vi "SPI API - SPI Simulation.vi"() -> ()   [LabVIEW 2014]
uses:
  Controls/Timing Characteristics.ctl
  Controls/Digital Data.ctl
  <vilib>/rvi/DesktopExecutionNode/Execution/niFpgaDEN_Execute.vi
  <vilib>/rvi/DesktopExecutionNode/DesktopExecutionNode.xnode
panel:
  in  "SPI PHY Settings":T1={"Divide Value"=10, "Transfer Length (bits)"=16, "CS Asserted Polarity"=FALSE, "Clock Polarity (CPOL)"=FALSE, "Clock Phase (CPHA)"=FALSE, "Lengthen MISO Setup"=FALSE, "Direction Change Bit"=0, "MOSI Starts as Output"=FALSE, "Tristatable MOSI"=FALSE}
  in  "Chip Select":u8
  in  "Engine Rate (MHz)":i32=120
  out "Data To Slave":u64 format="%b"
  out "Timing Characteristics":T2 {"tCL (ns)" format="%#_4g"; "tCH (ns)" format="%#_4g"; "tCSS (ns)" format="%#_4g"; "tCSH (ns)" format="%#_4g"; "tCSW (ns)" format="%#_4g"; "Actual Sample Rate (Hz)" format="%_4p"; "SCLK Frequency (Hz)" format="%#.2p"}
  in  "Pause":bool
  in  "Sample Rate (Hz)":u32=100000 format="%.0p"
  out "Digital Data":digitalwaveform(graph)
  in  "Data To Slave":u64 format="%x"
  in  "Stop":bool
  # "Operating Instructions\n1. For this VI to work, the FPGA must be in Simulation Mode.\n2. Set the 'Engine Rate' control value to match your FPGA SPI Engine loop rate.\n3. Select a sample rate to control how often the SPI message is transmitted.\n4. Run the VI and observe the Timing Characterstics to the right."
  # "Typical Timing Diagram"
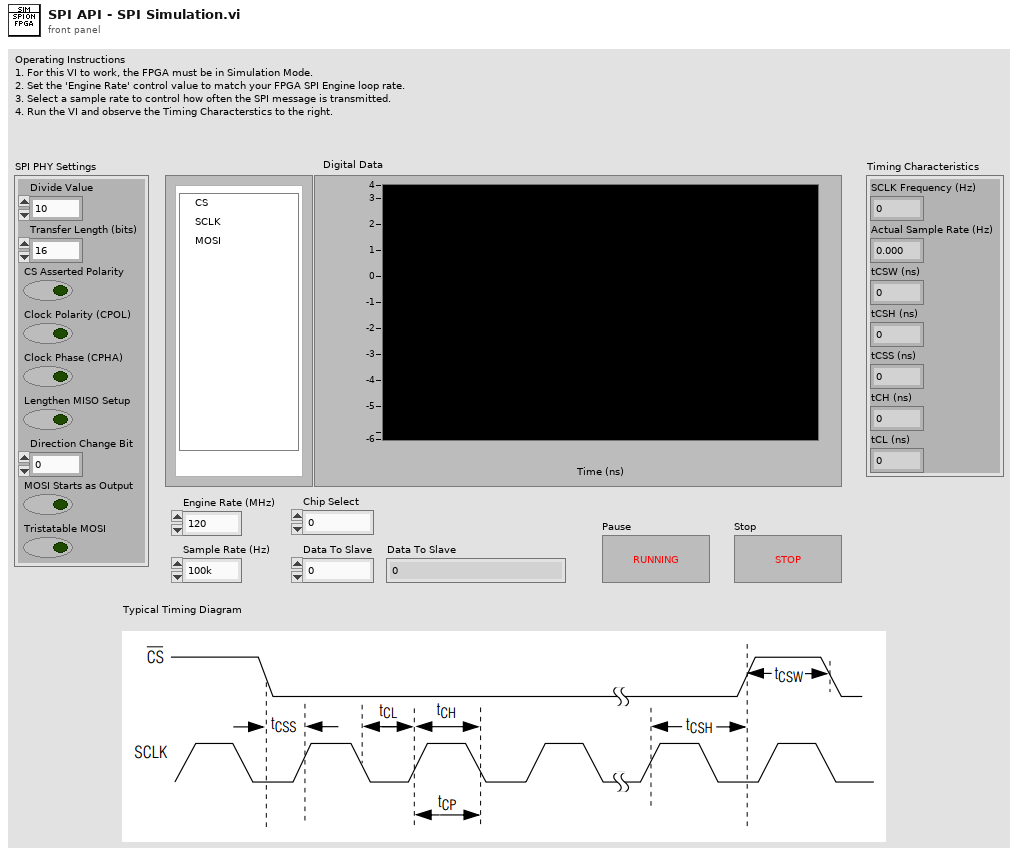
[diagram p1: front panel]
types:
  T1 = cluster{"Divide Value":u8, "Transfer Length (bits)":u8, "CS Asserted Polarity":bool, "Clock Polarity (CPOL)":bool, "Clock Phase (CPHA)":bool, "Lengthen MISO Setup":bool, "Direction Change Bit":u8, "MOSI Starts as Output":bool, "Tristatable MOSI":bool}
  T2 = typedef "Timing Characteristics.ctl" = cluster{"SCLK Frequency (Hz)":dbl, "Actual Sample Rate (Hz)":dbl, "tCSW (ns)":dbl, "tCSH (ns)":dbl, "tCSS (ns)":dbl, "tCH (ns)":dbl, "tCL (ns)":dbl}
  T3 = typedef "Digital Data.ctl" = cluster{"CS":bool, "SCLK":bool, "MISO":bool}
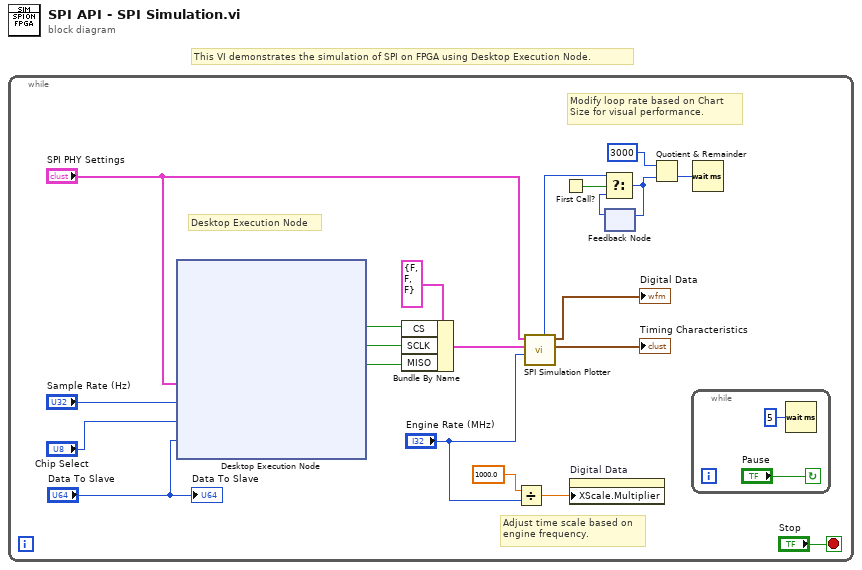
[diagram p0: block diagram]
diagram:
  # "This VI demonstrates the simulation of SPI on FPGA using Desktop Execution Node."
  n1 = while {
    stop <- "Stop" stop-if-true
    # "Adjust time scale based on\nengine frequency."
    # "Desktop Execution Node"
    # "Modify loop rate based on Chart\nSize for visual performance."
    n2 = xnode "Desktop Execution Node"("SPI PHY Settings"="SPI PHY Settings", "Sample Rate (Hz)"="Sample Rate (Hz)", "Chip Select"="Chip Select", "Tx"="Data To Slave") -> ("CS"=w7:bool, "SCLK"=w6:bool, "MOSI"=w5:bool)  [unwired: 1 in, 1 out]
    n3 = Bundle By Name(cluster=T3 {"CS"=FALSE, "SCLK"=FALSE, "MISO"=FALSE}, "CS"=w7, "SCLK"=w6, "MISO"=w5) -> (w14:T3)
    n4 = Divide(x=1000.0, y="Engine Rate (MHz)") -> (x/y=w8:dbl)
    n5 = call "SPI Simulation Plotter.vi"("Engine Clock Rate (MHz)"="Engine Rate (MHz)", "SPI Signals"=w14, "SPI PHY Settings"="SPI PHY Settings") -> ("Timing Characteristics"=→"Timing Characteristics":T2, "Digital Data"=→"Digital Data":digitalwaveform, "Chart Size"=w13:i32)  [unwired: 6 in]
    n6 = First Call?() -> (First Call?: T/F=w19:bool)
    n7 = property on="Digital Data" class="DigitalGraph (strict)"("XScale.Multiplier"=w8) -> ()  [unwired: 2 in, 2 out]
    n8 = feedback #1() -> (w18:i32)  [unwired: 1 in]
    n9 = Select(t=w13, s=w19, f=w18) -> (s? t:f=w17:i32)
    n10 = feedback-in #1(w17) -> ()
    n11 = Quotient & Remainder(x=u32 3000 ("ms per Command"), y=w17) -> (floor(x/y)=w15:u32)  [unwired: 1 out]
    n12 = while {
      stop <- "Pause" continue-if-true
      n13 = Wait (ms)(milliseconds to wait=u32 5) -> ()  [unwired: 1 out]
    }
    n14 = Wait (ms)(milliseconds to wait=w15) -> ()  [unwired: 1 out]
    "Data To Slave" <- "Data To Slave"
  }
